vi "GetMaxMin.vi"(8 "error in (no error)":errorcluster, 10 "Ignore Cal? (F)":bool, 11 "RTD in":refnum<class "RTD.lvclass">) -> (0 "error out":errorcluster, 1 "Min":cluster{"Value":dbl, "Text":string}, 2 "Max":cluster{"Value":dbl, "Text":string}, 3 "RTD out":refnum<class "RTD.lvclass">)   [LabVIEW 2018, in "Measurement Channels.lvlib" / "RTD.lvclass"]
uses:
  RTD.lvclass
  C:/Users/Jeff Tipps/Documents/DAQMan/source/Classes/Measurements/Class Channel/Channel.lvclass
  RTD.lvclass/RTD.ctl
  Class Channel/Read Scale.vi
  Class Channel/Read Offset.vi
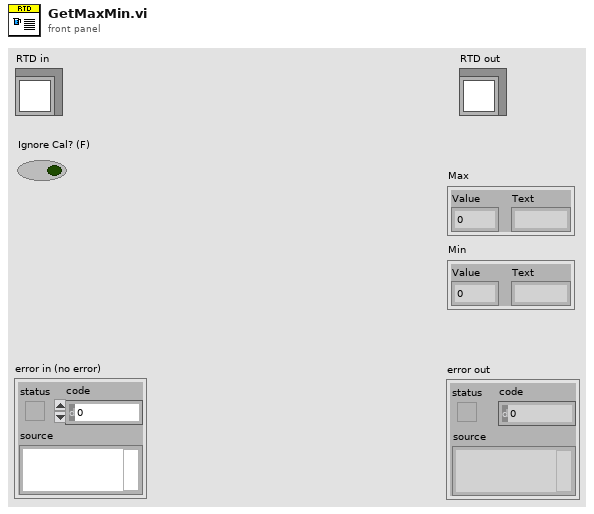
[diagram p1: front panel]
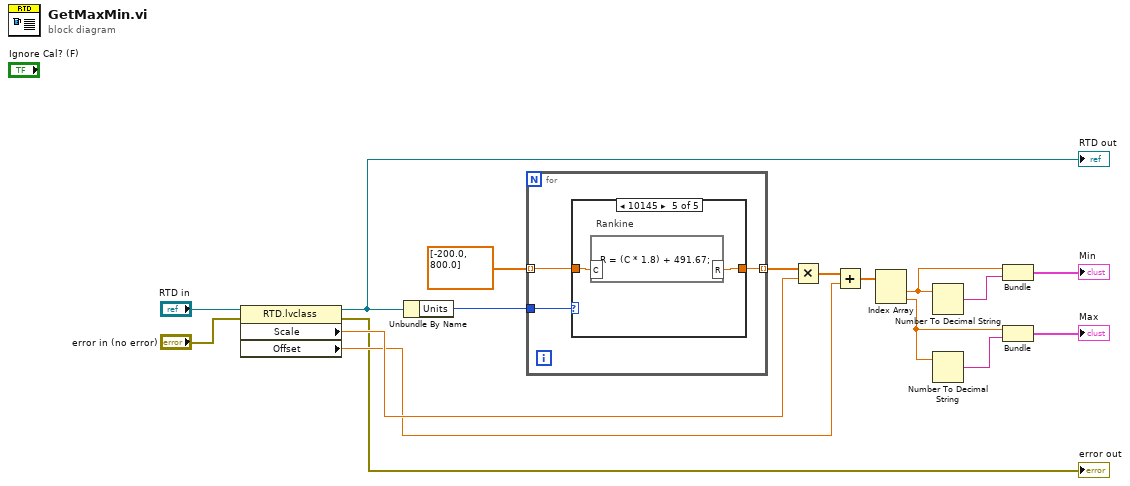
[diagram p0: block diagram]
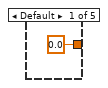
[diagram p2: hidden frame]
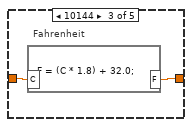
[diagram p4: hidden frame]
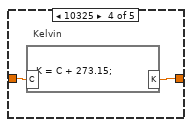
[diagram p5: hidden frame]
diagram:
  n1 = property class="RTD.lvclass"(reference="RTD in", error in="error in (no error)") -> (reference out=w7:refnum<class "RTD.lvclass">, error out=→"error out":errorcluster, "Scale"=w12:dbl, "Offset"=w11:dbl)
  "RTD out" <- w7
  n2 = Unbundle By Name(w7) -> ("Units"=w13:u16)
  n3 = for {
    tunnel: w13 -> [w20]
    tunnel: [w19] -> w16 mode=indexing
    tunnel: dbl[] [-200.0, 800.0] -> [w18] mode=indexing
    n4 = case shown="10145" w20 {
      tunnel: w18 -> [_ w22 w24 w26 w28]
      tunnel: [0.0 ("R") w22 w23 w25 w27] -> w19
      frame Default {
      }
      frame 10143 {
        # "Celsius"
      }
      frame 10144 {
        # "Fahrenheit"
        n5 = formula code="F = (C * 1.8) + 32.0;"("C"=w24) -> ("F"=w23:dbl)
      }
      frame 10325 {
        # "Kelvin"
        n6 = formula code="K = C + 273.15;"("C"=w26) -> ("K"=w25:dbl)
      }
      frame 10145 {
        # "Rankine"
        n7 = formula code="R = (C * 1.8) + 491.67;"("C"=w28) -> ("R"=w27:dbl)
      }
    }
  }
  n8 = Multiply(x=w16, y=w12) -> (x*y=w15:dbl[])
  n9 = Add(x=w15, y=w11) -> (x+y=w14:dbl[])
  n10 = Index Array(array=w14) -> (element #1=w6:dbl, element #2=w4:dbl)  [unwired: 2 in]
  n11 = Number To Decimal String(number=w6) -> (decimal integer string=w5:string)  [unwired: 1 in]
  n12 = Number To Decimal String(number=w4) -> (decimal integer string=w3:string)  [unwired: 1 in]
  n13 = Bundle(w6, w5) -> (→"Min":cluster{dbl, string})  [unwired: 1 in]
  n14 = Bundle(w4, w3) -> (→"Max":cluster{dbl, string})  [unwired: 1 in]
